vi "M06 Solar Cells tail.vi"(11 "EV3 in":T1) -> (3 "EV3 out":T1)   [LabVIEW 2016]
uses:
  <vilib>/NXT/Subs/LVHSConnector.ctl
  <vilib>/NXT/LegoClasses/BrickReference/BrickReference.lvclass
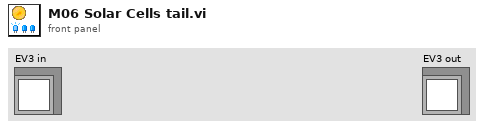
[diagram p1: front panel]
types:
  T1 = typedef "LVHSConnector.ctl" = refnum<class "BrickReference.lvclass">
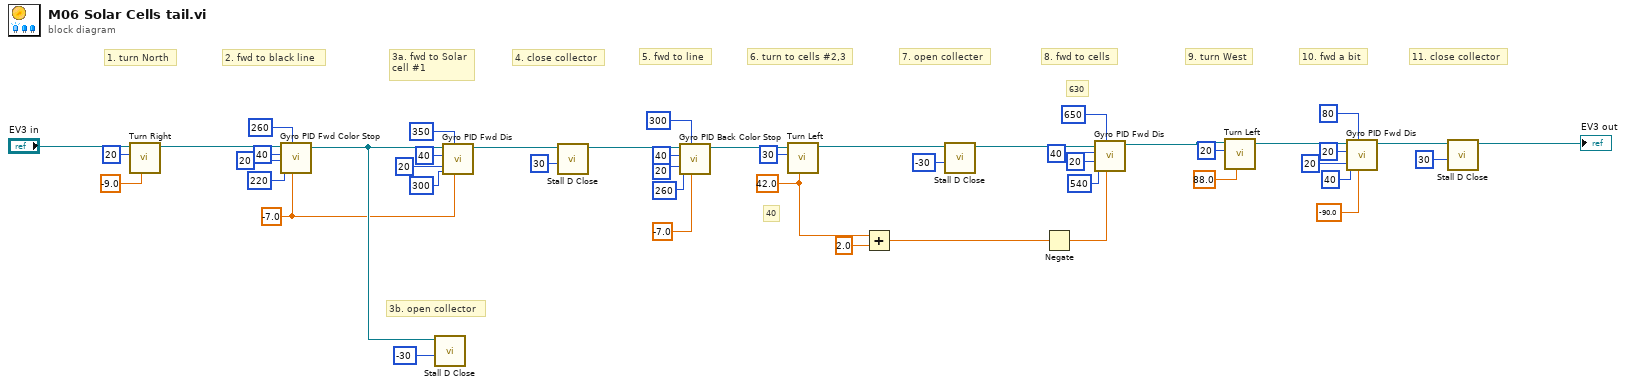
[diagram p0: block diagram]
diagram:
  w27 = sgl 42.0 ("Turning angle")
  w24 = sgl -7.0 ("Target angle")
  # "630"
  # "40"
  # "10. fwd a bit"
  # "9. turn West"
  # "5. fwd to line"
  # "4. close collector"
  # "7. open collecter"
  # "11. close collector"
  # "8. fwd to cells"
  # "6. turn to cells #2,3"
  # "3a. fwd to Solar\ncell #1"
  # "3b. open collector"
  # "2. fwd to black line"
  # "1. turn North"
  n1 = call "Turn Right.vi"("Turning angle"=sgl -9.0, "Motor B (right)"=i8 20, "EV3 in"="EV3 in") -> ("EV3 out"=w46:T1)  [unwired: 8 in]
  n2 = call "Gyro PID Fwd Color Stop.vi"("Target angle"=w24, "Threshold to Color"=260, "Threshold to slow"=220, "Min. speed"=20, "Max. speed"=40, "EV3 in"=w46) -> ("EV3 out"=w26:T1)  [unwired: 5 in]
  n3 = call "Stall D Close.vi"("Power"=i8 -30, "NXT/EV3"=w26) -> ()  [unwired: 9 in, 1 out]
  n4 = call "Gyro PID Fwd Dis.vi"("Target angle"=w24, "Threshold to stop"=350, "Threshold to slow"=300, "Min. speed"=20, "Max. speed"=40, "EV3 in"=w26) -> ("EV3 out"=w16:T1)  [unwired: 5 in]
  n5 = call "Stall D Close.vi"("Power"=i8 30, "NXT/EV3"=w16) -> ("NXT/EV3"=w22:T1)  [unwired: 9 in]
  n6 = call "Gyro PID Back Color Stop.vi"("Target angle"=sgl -7.0, "Threshold to Color"=300, "Threshold to slow"=260, "Min. speed"=20, "Max. speed"=40, "EV3 in"=w22) -> ("EV3 out"=w15:T1)  [unwired: 5 in]
  n7 = call "Turn Left.vi"("Turning angle"=w27, "Motor B (right)"=i8 30, "EV3 in"=w15) -> ("EV3 out"=w14:T1)  [unwired: 8 in]
  n8 = Add(x=w27, y=sgl 2.0) -> (x+y=w29:sgl)
  n9 = call "Stall D Close.vi"("Power"=i8 -30, "NXT/EV3"=w14) -> ("NXT/EV3"=w13:T1)  [unwired: 9 in]
  n10 = Negate(x=w29) -> (-x=w25:sgl)
  n11 = call "Gyro PID Fwd Dis.vi"("Target angle"=w25, "Threshold to stop"=650, "Threshold to slow"=540, "Min. speed"=20, "Max. speed"=40, "EV3 in"=w13) -> ("EV3 out"=w11:T1)  [unwired: 5 in]
  n12 = call "Turn Left.vi"("Turning angle"=sgl 88.0, "Motor B (right)"=i8 20, "EV3 in"=w11) -> ("EV3 out"=w8:T1)  [unwired: 8 in]
  n13 = call "Gyro PID Fwd Dis.vi"("Target angle"=sgl -90.0, "Threshold to stop"=80, "Threshold to slow"=40, "Min. speed"=20, "Max. speed"=20, "EV3 in"=w8) -> ("EV3 out"=w7:T1)  [unwired: 5 in]
  n14 = call "Stall D Close.vi"("Power"=i8 30, "NXT/EV3"=w7) -> ("NXT/EV3"=→"EV3 out":T1)  [unwired: 9 in]
